vi "ToString.vi"(8 "error in (no error)":errorcluster, 11 "Theory in":refnum<class "Theory.lvclass">) -> (0 "error out":errorcluster, 2 "String":string, 3 "Theory out":refnum<class "Theory.lvclass">)   [LabVIEW 2019, in "TestCase.lvlib" / "Theory.lvclass"]
doc: "Returns the string representation for this object."
uses:
  Theory.lvclass
  Theory.lvclass/Theory.ctl
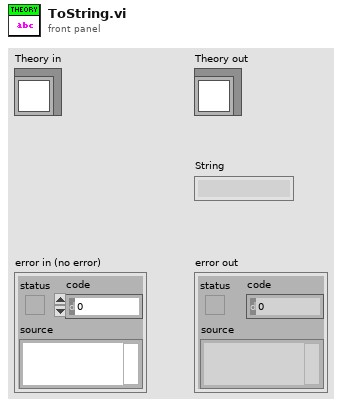
[diagram p1: front panel]
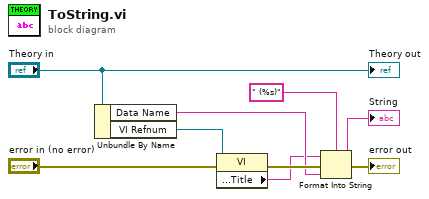
[diagram p0: block diagram]
diagram:
  n1 = Unbundle By Name("Theory in") -> ("Data Name"=w4:string, "VI Refnum"=w6:refnum<vi>)
  n2 = property class="VI"(reference=w6, error in="error in (no error)") -> (error out=w8:errorcluster, "Front Panel.Title"=w1:string)  [unwired: 1 out]
  n3 = Format Into String(format string=" (%s)", initial string=w1, error in=w8, w4) -> (resulting string=→"String":string, error out=→"error out":errorcluster)
  "Theory out" <- "Theory in"
